vi "Set_Pigeon_Status_Period.vi"(8 "error in (no error)":errorcluster) -> (0 "error out":errorcluster)   [LabVIEW 2020]
uses:
  <vilib>/Rock Robotics/WPI/ThirdParty/Phoenix-LabVIEW/Pigeon IMU/CTRE_PigeonIMU_DeviceRef.ctl
  <vilib>/Rock Robotics/WPI/ThirdParty/Phoenix-LabVIEW/Pigeon IMU/CTRE_PigeonIMU_ConnectionType.ctl
  <vilib>/Rock Robotics/WPI/ThirdParty/Phoenix-LabVIEW/Pigeon IMU/CTRE_PigeonIMU_StatusFrameRate.ctl
  Status Config Array.ctl
  STATUS_Period.ctl
  8bffcf12-d87b-4679-b93c-e69f5877cc70.vi
  <vilib>/Comparison/Equal/Equal Functor/Equal Functor.lvclass
panel:
  in  "Status Config Array":T1=[{"Status Frame Enum"=270336, "STATUS_Period"=240}] {"Status Frame Enum" items=["CondStatus_1_General"=270336, "CondStatus_9_SixDeg_YPR"=270848, "CondStatus_6_SensorFusion"=270656, "CondStatus_11_GyroAccum"=270976, "CondStatus_2_GeneralCompass"=270400, "CondStatus_3_GeneralAccel"=270464, "CondStatus_10_SixDeg_Quat"=270912, "RawStatus_4_Mag"=265408, "BiasedStatus_2_Gyro"=269376, "BiasedStatus_4_Mag"=269504, "BiasedStatus_6_Accel"=269632]; "STATUS_Period" items=["Low (240ms)"=240, "Medium (50ms)"=50, "High (10ms)"=10]}
  in  "Status Frame Enum":T2=270336 items=["CondStatus_1_General"=270336, "CondStatus_9_SixDeg_YPR"=270848, "CondStatus_6_SensorFusion"=270656, "CondStatus_11_GyroAccum"=270976, "CondStatus_2_GeneralCompass"=270400, "CondStatus_3_GeneralAccel"=270464, "CondStatus_10_SixDeg_Quat"=270912, "RawStatus_4_Mag"=265408, "BiasedStatus_2_Gyro"=269376, "BiasedStatus_4_Mag"=269504, "BiasedStatus_6_Accel"=269632]
  out "PigeonIMUDevRef":T4={"DeviceStatus"={"status"=FALSE, "code"=0, "source"=""}, "Device Number"=0, "Type"=352321536, "Device ID"=0, "Handle"=0, "UsageFrame"=0, "Library Path"=path ""} {"Type" items=["CAN"=352321536, "TalonSRX"=33554432]}
  in  "PigeonIMUDevRef":T4={"DeviceStatus"={"status"=FALSE, "code"=0, "source"=""}, "Device Number"=0, "Type"=352321536, "Device ID"=0, "Handle"=0, "UsageFrame"=0, "Library Path"=path ""} {"Type" items=["CAN"=352321536, "TalonSRX"=33554432]}
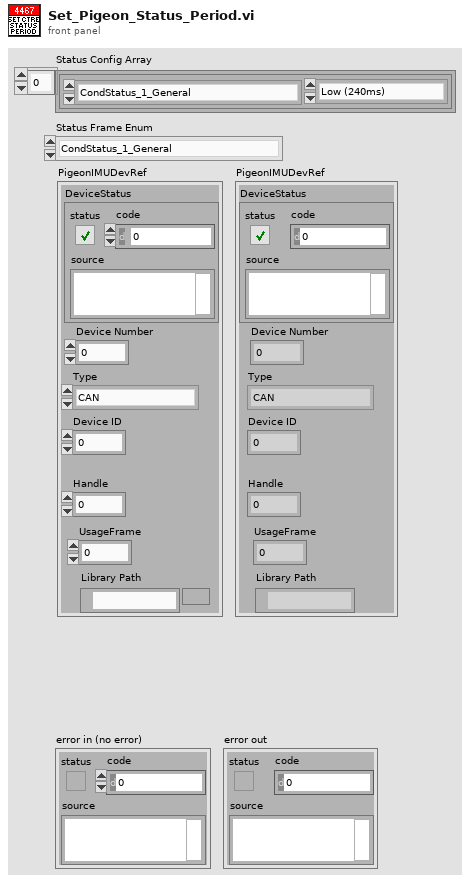
[diagram p1: front panel]
types:
  T1 = typedef "Status Config Array.ctl" = cluster{"Status Frame Enum":T2, "STATUS_Period":T3}[]
  T2 = typedef "CTRE_PigeonIMU_StatusFrameRate.ctl" = u32
  T3 = typedef "STATUS_Period.ctl" = i32
  T4 = typedef "CTRE_PigeonIMU_DeviceRef.ctl" = cluster{"DeviceStatus":errorcluster, "Device Number":u8, "Type":T5, "Device ID":u32, "Handle":u64, "UsageFrame":u32, "Library Path":path}
  T5 = typedef "CTRE_PigeonIMU_ConnectionType.ctl" = u32
  T6 = typedef "LVStringsAndValuesArrayTypeDef_U32.ctl" = cluster{"String":string, "Value":u32}[]
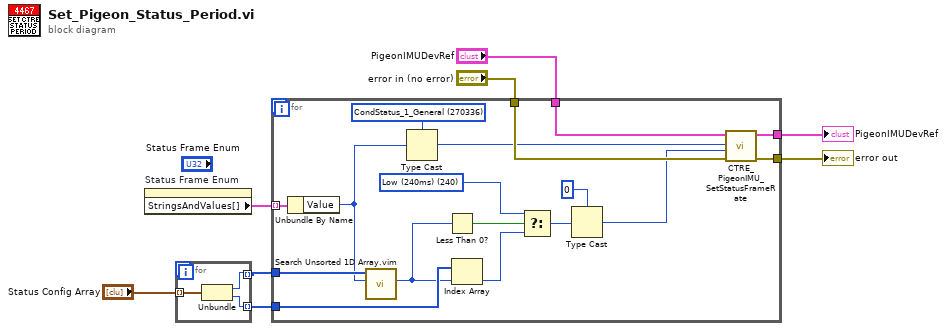
[diagram p0: block diagram]
diagram:
  n1 = property on="Status Frame Enum" class="Ring (strict)"() -> ("StringsAndValues[]"=w7:T6)  [unwired: 2 in, 2 out]
  n2 = for {
    tunnel: "Status Config Array" -> [w9] mode=indexing
    tunnel: [w11] -> w5 mode=indexing
    tunnel: [w10] -> w4 mode=indexing
    n3 = Unbundle(w9) -> ("Status Frame Enum"=w11:T2, "STATUS_Period"=w10:T3)
  }
  n4 = for {
    tunnel: [w28] -> w2
    tunnel: [w27] -> w8
    tunnel: w7 -> [w21] mode=indexing
    tunnel: w5 -> [w26]
    tunnel: w4 -> [w25]
    tunnel: "error in (no error)" -> [w20]
    tunnel: "PigeonIMUDevRef" -> [w16]
    w12 = T3 240 items=["Low (240ms)"=240, "Medium (50ms)"=50, "High (10ms)"=10] ("STATUS_Period")
    w15 = T2 270336 items=["CondStatus_1_General"=270336, "CondStatus_9_SixDeg_YPR"=270848, "CondStatus_6_SensorFusion"=270656, "CondStatus_11_GyroAccum"=270976, "CondStatus_2_GeneralCompass"=270400, "CondStatus_3_GeneralAccel"=270464, "CondStatus_10_SixDeg_Quat"=270912, "RawStatus_4_Mag"=265408, "BiasedStatus_2_Gyro"=269376, "BiasedStatus_4_Mag"=269504, "BiasedStatus_6_Accel"=269632] ("StatusFrame")
    n5 = Unbundle By Name(w21) -> ("Value"=w17:u32)
    n6 = call "Search Unsorted 1D Array.vim"("element"=w17, "unsorted 1D array"=w26) -> ("index of element"=w24:i32)  [unwired: 9 in]
    n7 = Type Cast(type=w15, x=w17) -> (*(type *) &x=w14:T2)
    n8 = Less Than 0?(x=w24) -> (x < 0?=w23:bool)
    n9 = Index Array(array=w25, index=w24) -> (element=w22:T3)
    n10 = Select(t=w12, s=w23, f=w22) -> (s? t:f=w19:T3)
    n11 = Type Cast(type=i16 0, x=w19) -> (*(type *) &x=w13:i16)
    n12 = call <vilib>:"CTRE_PigeonIMU_SetStatusFrameRate.vi"("error in (no error)"=w20, "Period (ms)"=w13, "StatusFrame"=w14, "PigeonIMUDevRef"=w16) -> ("error out"=w27:errorcluster, "PigeonIMUDevRef"=w28:T4)  [unwired: 6 in]
  }
  "error out" <- w8
  "PigeonIMUDevRef" <- w2
